vi "FTW-ActorRef-SendMessage-Shutdown.vi"(0 "Actor Reference":refnum<class "FTW-ActorReference.lvclass">, 11 "error in":errorcluster) -> (4 "Actor Reference out":refnum<class "FTW-ActorReference.lvclass">, 15 "error out":errorcluster)   [LabVIEW 2012, in "FTW-ActorReference.lvclass"]
uses:
  FTW-ActorReference.lvclass
panel:
  # "Inputs"
  # "Outputs"
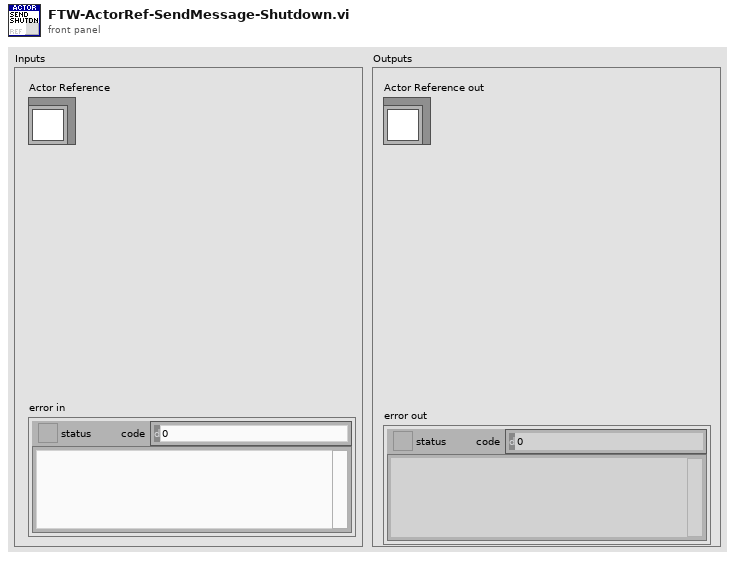
[diagram p1: front panel]
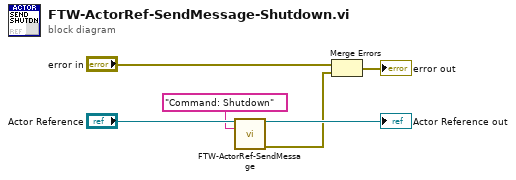
[diagram p0: block diagram]
diagram:
  n1 = call "FTW-ActorRef-SendMessage.vi"("Actor Reference"="Actor Reference", "Message"="Command: Shutdown") -> ("Actor Reference out"=→"Actor Reference out":refnum<class "FTW-ActorReference.lvclass">, "error out"=w1:errorcluster)  [unwired: 12 in]
  n2 = Merge Errors("error in", w1) -> (→"error out":errorcluster)
